vi "IPS Reply to PGSQL.vi"(8 "error in (no error)":errorcluster, 10 "Response":T1) -> (0 "error out":errorcluster)   [LabVIEW 2016, in "Instrument.Oxford1820.lvclass"]
uses:
  Instrument.Oxford1820.lvclass
  <instrlib>/Mercury iXX/Public/Controls/Response String.ctl
  <userlib>/LevyLab/postgreSQL-timescaleDB/Data.PG/Data.PGSQL.lvclass
  <instrlib>/Mercury iXX/Mercury iXX.lvlib
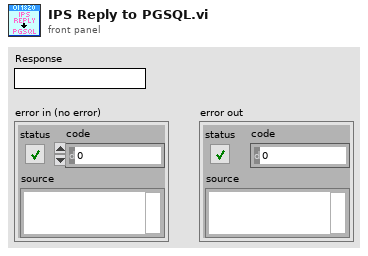
[diagram p1: front panel]
types:
  T1 = typedef "Mercury iXX.lvlib/Response String.ctl" = string
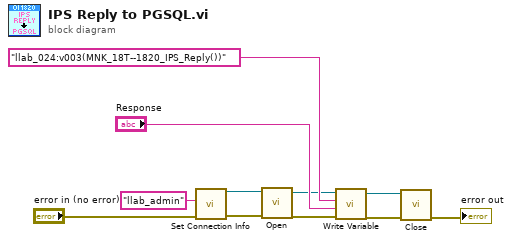
[diagram p0: block diagram]
diagram:
  n1 = call <userlib>:"Set Connection Info.vi"("username"="llab_admin", "error in (no error)"="error in (no error)") -> ("Data.PG out"=w7:refnum<class "Data.PGSQL.lvclass">, "error out"=w6:errorcluster)  [unwired: 7 in]
  n2 = call-dynamic "Open.vi"("error in (no error)"=w6, "Data.PG in"=w7) -> ("error out"=w4:errorcluster, "Data.PG out"=w5:refnum<class "Data.PGSQL.lvclass">)  [unwired: 8 in]
  n3 = call <userlib>:"Write Variable.vi"("error in (no error)"=w4, "Data"="Response", "variable"="llab_024:v003(MNK_18T--1820_IPS_Reply())", "Data.PG in"=w5) -> ("error out"=w2:errorcluster, "Data.PG out"=w3:refnum<class "Data.PGSQL.lvclass">)  [unwired: 5 in, 1 out]
  n4 = call-dynamic "Close.vi"("error in (no error)"=w2, "Data.PG in"=w3) -> ("error out"=→"error out":errorcluster)  [unwired: 8 in, 1 out]
